vi "Read Analogue.vi"(8 "error in (no error)":errorcluster, 11 "ACIR Instrument":refnum<class "ACIR Instrument.lvclass">) -> (0 "error out":errorcluster, 2 "Waveforms":waveform(dbl)[](array[waveform]), 3 "ACIR Instrument out":refnum<class "ACIR Instrument.lvclass">)   [LabVIEW 2025, in "ACIR.lvlib" / "ACIR Instrument.lvclass"]
uses:
  ACIR Instrument.lvclass
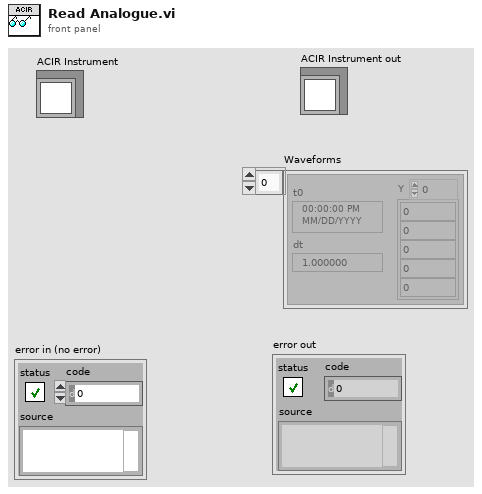
[diagram p1: front panel]
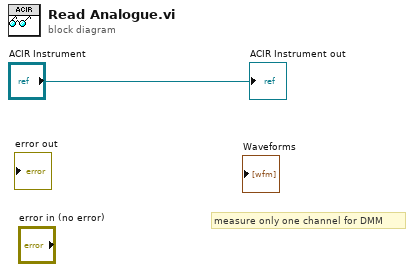
[diagram p0: block diagram]
diagram:
  # "measure only one channel for DMM"
  "ACIR Instrument out" <- "ACIR Instrument"
